vi "Keithley6487_example.vi"(11 "VISA resource name":refnum<visa-resource-name>) -> ()   [LabVIEW 2016]
panel:
  out "error out":errorcluster
  in  "Stop":bool
  out "output":dbl
  in  "range (auto)":T1(ring)
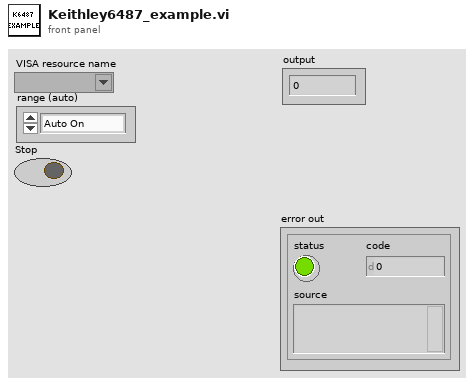
[diagram p1: front panel]
types:
  T1 = enum16{"Auto On", "2e-9", "2e-8", "2e-7", "2e-6", "2e-5", "2e-4", "2e-3", "2e-2"}
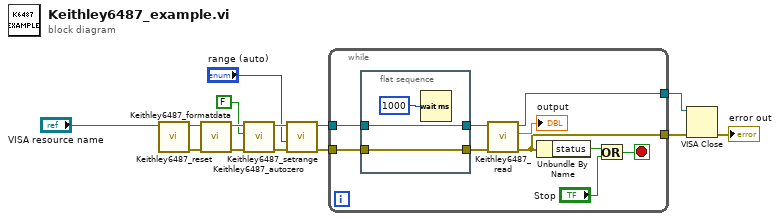
[diagram p0: block diagram]
diagram:
  n1 = call "Keithley6487_reset.vi"("VISA resource name"="VISA resource name") -> ("error out"=w13:errorcluster, "VISA resource name out"=w10:refnum<visa-resource-name>)  [unwired: 9 in]
  n2 = call "Keithley6487_formatdata.vi"("error in (no error)"=w13, "VISA resource name"=w10) -> ("error out"=w12:errorcluster, "VISA resource name out"=w9:refnum<visa-resource-name>)  [unwired: 8 in]
  n3 = call "Keithley6487_autozero.vi"("error in (no error)"=w12, "Autozero"=FALSE, "VISA resource name"=w9) -> ("error out"=w11:errorcluster, "VISA resource name out"=w8:refnum<visa-resource-name>)  [unwired: 7 in]
  n4 = call "Keithley6487_setrange.vi"("error in (no error)"=w11, "Enum"="range (auto)", "VISA resource name"=w8) -> ("error out"=w6:errorcluster, "VISA resource name out"=w7:refnum<visa-resource-name>)  [unwired: 7 in]
  n5 = while {
    tunnel: w7 -> [w24]
    tunnel: w6 -> [w22]
    tunnel: [w16] -> w2
    tunnel: [w15] -> w3
    stop <- w17 stop-if-true
    n6 = flat-sequence {
      tunnel: [w26] -> w23
      tunnel: w24 -> [w26]
      tunnel: [w25] -> w21
      tunnel: w22 -> [w25]
      frame #0 {
        n7 = Wait (ms)(milliseconds to wait=u32 1000) -> ()  [unwired: 1 out]
      }
    }
    n8 = call "Keithley6487_read.vi"("error in (no error)"=w21, "VISA resource name"=w23) -> ("error out"=w15:errorcluster, "output"=→"output":dbl, "VISA resource name out"=w16:refnum<visa-resource-name>)  [unwired: 7 in]
    n9 = Unbundle By Name(w15) -> ("status"=w19:bool)
    n10 = Or(x=w19, y="Stop") -> (x .or. y?=w17:bool)
  }
  n11 = VISA Close(VISA resource name=w2, error in (no error)=w3) -> (error out=→"error out":errorcluster)
